vi "Determinar_FT.vi"() -> ()   [LabVIEW 2013]
uses:
  <vilib>/addons/Control Design/_Utility/Model Viewer.llb/Model Viewer SubVI/cd_Draw Transfer Function Equation (TF).vi
  <vilib>/addons/Control Design/_Time Response Analysis/Time Response.llb/Time Response subVI/cd_Step Response (Transfer Function).vi
  <vilib>/imath/engines/lvmath2/RunTimeEngine/ErrorHandling/NIMS_Finalize Error.vi
  <vilib>/imath/engines/lvmath2/RunTimeEngine/Managers/WorkSpace/UID Generator.vi
  <vilib>/imath/engines/lvmath2/RunTimeEngine/Managers/SymbolTable/Clear UID.vi
  <vilib>/imath/engines/lvmath2/RunTimeEngine/NodeEndStatement/NIMS_NodeEndStatement_Output.vi
  <instcachedir>/0/NIMS_NodeEndStatement_Output_53EC0D466D134D7ABD903AC30B43404B.lvgen/NIMS_NodeEndStatement_Output_53EC0D466D134D7ABD903AC30B43404B_001.vi
  <instcachedir>/0/NIMS_NodeEndStatement_Output_53EC0D466D134D7ABD903AC30B43404B.lvgen/NIMS_NodeEndStatement_Output_53EC0D466D134D7ABD903AC30B43404B_011.vi
  <instcachedir>/0/NIMS_NodeEndStatement_Output_53EC0D466D134D7ABD903AC30B43404B.lvgen/NIMS_NodeEndStatement_Output_53EC0D466D134D7ABD903AC30B43404B_010.vi
  <vilib>/imath/engines/lvmath2/RunTimeEngine/BuiltInFunctions/close/NIMS_close(Enums).vi
  <vilib>/imath/engines/lvmath2/RunTimeEngine/IndexRead/NIMS V(R2).vi
  <instcachedir>/0/NIMS V(R2)_C76619605A0E4E9F8B2FA9389712AC47.lvgen/NIMS V(R2)_C76619605A0E4E9F8B2FA9389712AC47_000.vi
  <vilib>/imathl/engines/lvmath/Functions/Error Handling/Create Error.vi
  <vilib>/imath/engines/lvmath2/RunTimeEngine/BuiltInFunctions/size/NIMS_I32Row=size(GRow).vi
  <instcachedir>/0/NIMS_I32Row=size(GRow)_E5C05C6B13124B29B774CC4F993D3C59.lvgen/NIMS_I32Row=size(GRow)_E5C05C6B13124B29B774CC4F993D3C59_000.vi
  <vilib>/imath/engines/lvmath2/RunTimeEngine/IndexRead/NIMS V(S).vi
  <instcachedir>/0/NIMS V(S)_0488751826AF41519A22953C041130DC.lvgen/NIMS V(S)_0488751826AF41519A22953C041130DC_002.vi
  <vilib>/imath/engines/lvmath2/RunTimeEngine/RangeToken/NIMS_Range.vi
  <instcachedir>/0/NIMS_Range_7481B155BEE341ECA0F59DDB444E2C09.lvgen/NIMS_Range_7481B155BEE341ECA0F59DDB444E2C09_000.vi
  <vilib>/imath/engines/lvmath2/RunTimeEngine/IndexReplace/NIMS V(S)=M.vi
  <instcachedir>/0/NIMS V(S)=M_96830950E3C3491086A4BED53A3AB9F4.lvgen/NIMS V(S)=M_96830950E3C3491086A4BED53A3AB9F4_001.vi
  <vilib>/imath/engines/lvmath2/RunTimeEngine/BuiltInFunctions/max/1 input/NIMS_max(RV).vi
  <instcachedir>/0/NIMS_max(RV)_237633DB1D604D5BA7001287DF3C7957.lvgen/NIMS_max(RV)_237633DB1D604D5BA7001287DF3C7957_000.vi
  <instcachedir>/0/NIMS V(S)_0488751826AF41519A22953C041130DC.lvgen/NIMS V(S)_0488751826AF41519A22953C041130DC_000.vi
  <vilib>/imath/engines/lvmath2/RunTimeEngine/BuiltInFunctions/findnz/NIMS_[1o]_findnz(GRowV).vi
  <instcachedir>/0/NIMS_[1o]_findnz(GRowV)_A907680C39E74AF18CBD76E991AC1137.lvgen/NIMS_[1o]_findnz(GRowV)_A907680C39E74AF18CBD76E991AC1137_000.vi
  <vilib>/imath/engines/lvmath/Plug In/Control Design/BuiltInFunctions/tf/NIMS_CD_tf(num,den,Ts).vi
  <vilib>/imath/engines/lvmath/Plug In/Control Design/BuiltInFunctions/multmx/NIMS_CD_multmx(K,TF).vi
  <vilib>/imath/engines/lvmath/Plug In/Control Design/BuiltInFunctions/multmx/NIMS_CD_multmx(TF,TF).vi
  <vilib>/imath/engines/lvmath/Plug In/Control Design/BuiltInFunctions/plus/NIMS_CD_plus(TF,K).vi
  <vilib>/imath/engines/lvmath/Functions/Error Handling/MergeErrorsWrapper.vi
  <vilib>/addons/Control Design/_Time Response Analysis/NI_CD_Time Response.lvlib
  <vilib>/addons/Control Design/_Utility/NI_CD_Model Viewer.lvlib
  <vilib>/imath/engines/lvmath2/RunTimeEngine/Managers/SymbolTable/NIMS_WorkSpace.lvlib
panel:
  out "Tamb":dbl=25.85494094122024
  out "Tau":dbl=55.42957331762942
  out "Theta":dbl=42.90610311044488
  out "K":dbl=0.5791232122189154
  out "Resposta degrau, FT determinada":cluster{"time":dbl[], dbl[]}[](graph)
  out "FT sem atraso":picture
  out "Finished":bool
  in  "Enable_computing":bool
  in  "Time Target (s)":dbl=300.0
  out "Waveform INPUT":dynamicdata(graph)=[{"t0"=timestamp(3771854592.7277975 s since 1904-01-01), "dt"=1.0, "Y"=[-4.527297247023809], "attributes"=variant("NI_ChannelName"=variant(string "Filtered"))}]
  out "Elapsed Time (s)":dbl
  in  "Determinar FT":bool
  in  "stop":bool
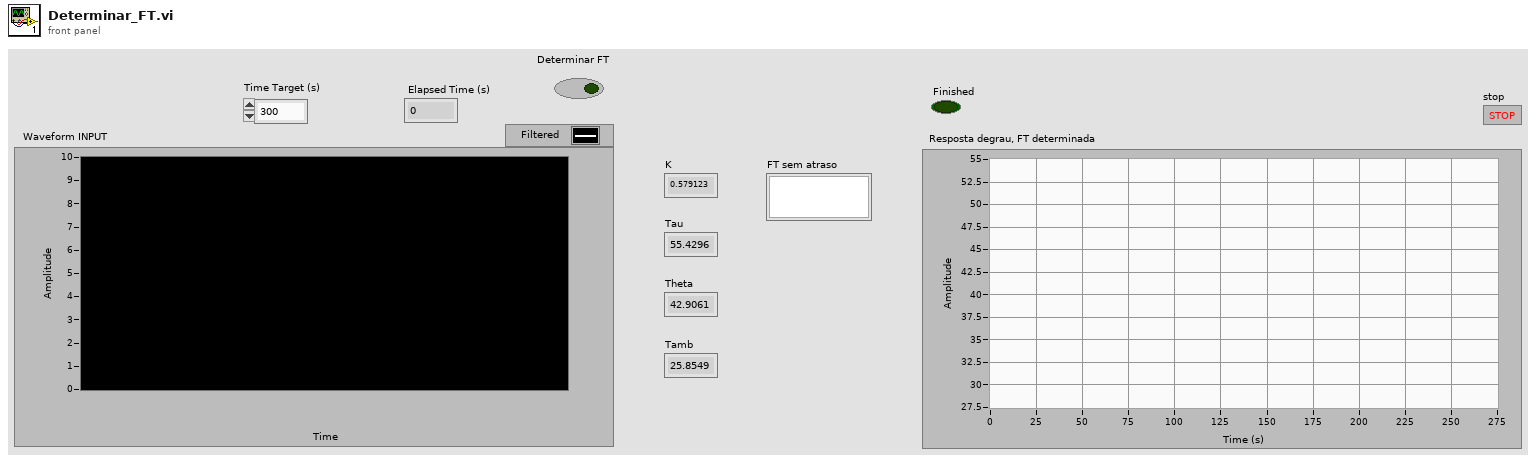
[diagram p1: front panel]
types:
  T1 = typedef "NI_LinSys_Model Typedefs.lvlib/CD Transfer Function Model (MIMO).ctl" = cluster{"properties":T2, "transfer function(s)":T3[][]}
  T2 = typedef "NI_LinSys_Model Typedefs.lvlib/CD General Elements.ctl" = cluster{"Model name":string, "Input names":string[], "Output names":string[], "Input Delays":dbl[], "Output Delays":dbl[], "Sampling Time":dbl, "Notes":string}
  T3 = typedef "NI_LinSys_Model Typedefs.lvlib/CD Transfer Function Model (SISO).ctl" = cluster{"Numerator":dbl[], "Denominator":dbl[], "delay":dbl}
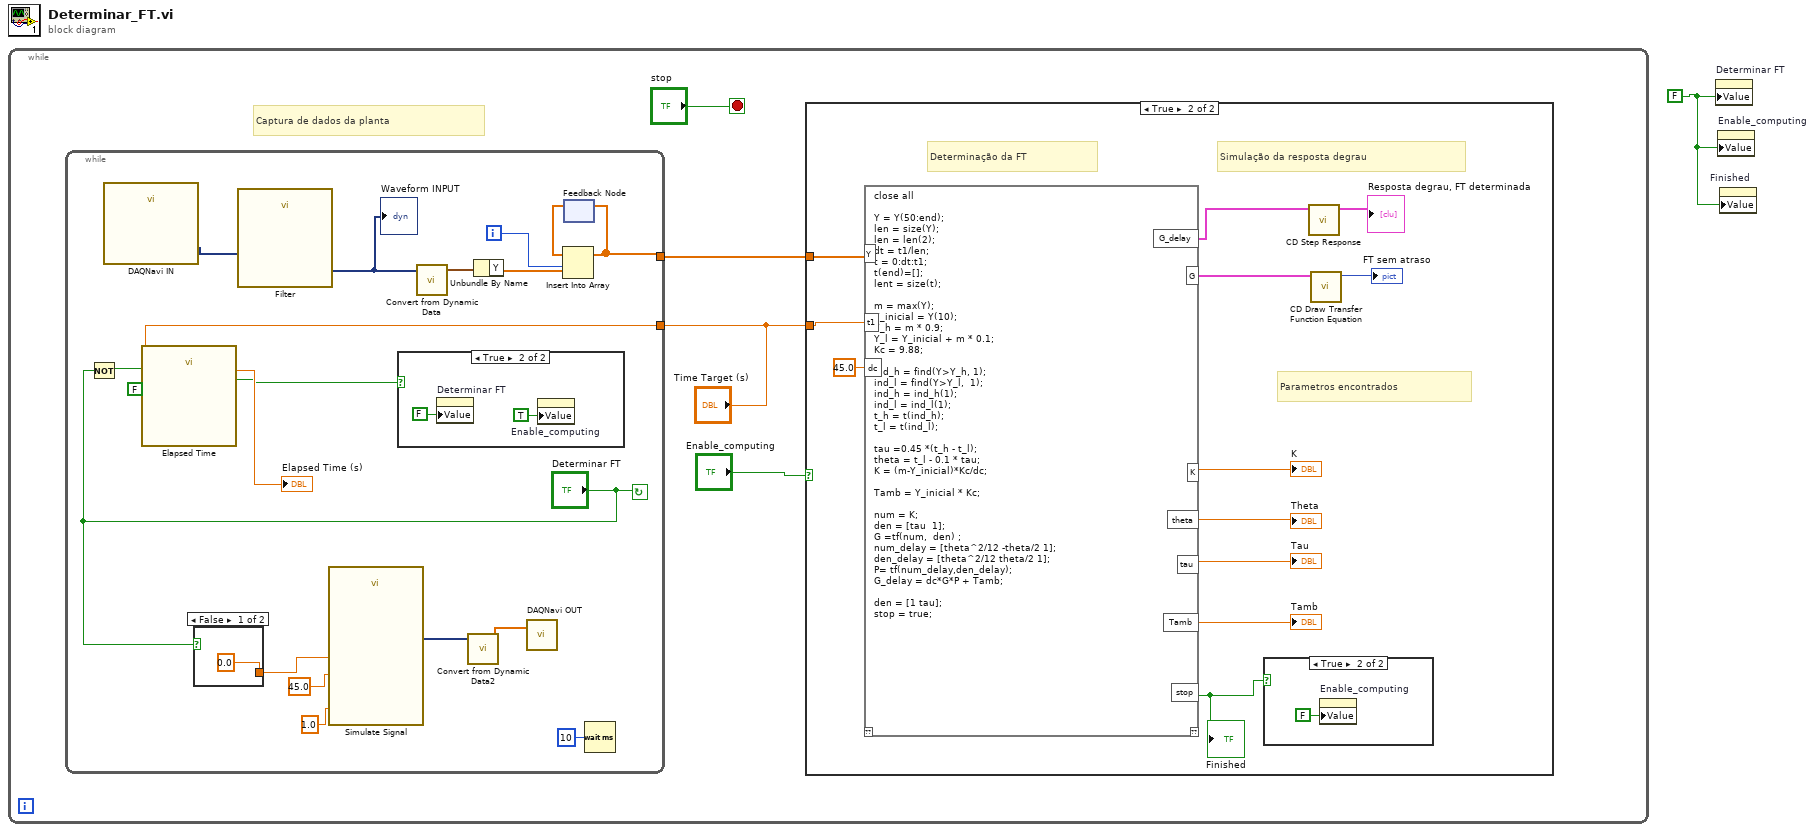
[diagram p0: block diagram]
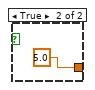
[diagram p4: hidden frame]
diagram:
  w1 = FALSE ("Enable_computing")
  n1 = while {
    stop <- "stop" stop-if-true
    # "Captura de dados da planta"
    n2 = while {
      tunnel: [w454] -> w4
      tunnel: "Time Target (s)" -> [w448]
      i -> [w449]
      stop <- "Determinar FT" continue-if-true
      n3 = Not(x="Determinar FT") -> (.not. x?=w446:bool)
      n4 = call "DAQNavi IN"() -> ("data out(DDT)"=w450:dynamicdata)  [unwired: 26 in, 1 out]
      n5 = call "Elapsed Time"("Time Target (s)"=w448, "Reset"=w446, "Auto Reset"=FALSE) -> ("Elapsed Time (s)"=→"Elapsed Time (s)":dbl, "Time has Elapsed"=w452:bool)  [unwired: 2 in, 13 out]
      n6 = case shown="False" "Determinar FT" {
        tunnel: [0.0 ("Amplitude") 5.0 ("Amplitude")] -> w440
        frame False {
        }
        frame True {
        }
      }
      n7 = call "Filter"("Signal"=w450) -> ("Filtered Signal"=w451:dynamicdata)  [unwired: 9 in, 1 out]
      "Waveform INPUT" <- w451
      n8 = call "Simulate Signal"("Duty Cycle (%)"=45.0, "Frequency"=1.0, "Amplitude"=w440) -> ("Square"=w442:dynamicdata)  [unwired: 11 in, 1 out]
      n9 = case shown="True" w452 {
        frame False {
        }
        frame True {
          n10 = property on="Determinar FT" class="Bool (strict)"("Value"=FALSE ("Enable_capture")) -> ()  [unwired: 2 in, 2 out]
          n11 = property on="Enable_computing" class="Bool (strict)"("Value"=TRUE ("Enable_computing")) -> ()  [unwired: 2 in, 2 out]
        }
      }
      n12 = call "Convert from Dynamic Data"("Dynamic Data Type"=w451) -> ("Waveform"=w456:waveform(dbl))  [unwired: 3 in]
      n13 = call "Convert from Dynamic Data2"("Dynamic Data Type"=w442) -> ("Array"=w443:dbl[])  [unwired: 3 in]
      n14 = Unbundle By Name(w456) -> ("Y"=w447:dbl[])
      n15 = call "DAQNavi OUT"("dataIn(U8Array)"=w443) -> ()  [unwired: 26 in, 1 out]
      n16 = feedback #1() -> (w455:dbl[])  [unwired: 1 in]
      n17 = Insert Into Array(array=w455, index=w449, new element=w447) -> (w454:dbl[])
      n18 = feedback-in #1(w454) -> ()
      n19 = Wait (ms)(milliseconds to wait=u32 10) -> ()  [unwired: 1 out]
    }
    n20 = case shown="True" "Enable_computing" {
      tunnel: w4 -> [_ w12]
      tunnel: "Time Target (s)" -> [_ w11]
      frame False {
      }
      frame True {
        # "Parametros encontrados"
        # "Simulação da resposta degrau"
        # "Determinação da FT"
        n21 = mathscript code="close all\n\nY = Y(50:end);\nlen = size(Y);\nlen = len(2); \ndt = t1/len;\nt = 0:dt:t1;\nt(end)=[];\nlent = size(t);\n\nm = max(Y);\nY_inicial = Y(10);\nY_h = m * 0.9;\nY_l = Y_inicial + m * 0.1;\nKc = 9.88;\n\nind_h = find(Y>Y_h, 1);\nind_l = find(Y>Y_l,  1);\nind_h = ind_h(1);\nind_l = ind_l(1);\nt_h = t(ind_h);\nt_l = t(ind_l);\n\ntau =0.45 *(t_h - t_l);\ntheta = t_l - 0.1 * tau;\nK = (m-Y_inicial)*Kc/dc;\n\nTamb = Y_inicial * Kc;\n\nnum = K;\nden = [tau  1];\nG =tf(num,  den) ;\nnum_delay = [theta^2/12 -theta/2 1];\nden_delay = [theta^2/12 theta/2 1];\nP= tf(num_delay,den_delay);\nG_delay = dc*G*P + Tamb;\n\nden = [1 tau];\nstop = true;"("Y"=w12, "t1"=w11, "dc"=45.0) -> ("G_delay"=w13:T1, "G"=w14:T1, "theta"=→"Theta":dbl, "stop"=w15:bool, "Tamb"=→"Tamb":dbl, "K"=→"K":dbl, "tau"=→"Tau":dbl)  [unwired: 1 in, 1 out]
        "Finished" <- w15
        n22 = case shown="True" w15 {
          frame False {
          }
          frame True {
            n23 = property on="Enable_computing" class="Bool (strict)"("Value"=FALSE ("Enable_computing")) -> ()  [unwired: 2 in, 2 out]
          }
        }
        n24 = call-poly <vilib>:"CD Step Response.vi"("Transfer Function Model"=w13) -> ("Step Response Graph"=→"Resposta degrau, FT determinada":cluster{"time":dbl[], dbl[]}[])  [unwired: 8 in, 2 out]
        n25 = call-poly <vilib>:"CD Draw Transfer Function Equation.vi"("Transfer Function Model"=w14) -> ("Equation"=→"FT sem atraso":picture)  [unwired: 8 in, 2 out]
      }
    }
  }
  n26 = property on="Determinar FT" class="Bool (strict)"("Value"=w1) -> ()  [unwired: 2 in, 2 out]
  n27 = property on="Enable_computing" class="Bool (strict)"("Value"=w1) -> ()  [unwired: 2 in, 2 out]
  n28 = property on="Finished" class="Bool (strict)"("Value"=w1) -> ()  [unwired: 2 in, 2 out]
